vi "FPGA_controller.vi"() -> ()   [LabVIEW 2017]
uses:
  <vilib>/rvi/Emulation/niFpgaGetClockAttributes.vi
  <vilib>/rvi/Emulation/niFpgaSctlEmulationGetInTimedLoop.vi
  <vilib>/rvi/Emulation/niFpgaEmulationReportErrorSimple.vi
  <vilib>/rvi/eio/common/nirviEmuTemplateMethod_errors.vi
  <vilib>/rvi/Emulation/niFpgaCriticalErrorInLSC.vi
  <vilib>/eio/EIONode/EIONode.xnode
panel:
  out "Translated":i16
  out "VALID":bool
  in  "m_first u2":fxp<+/-,64,32>=-0.8999999999068677 format="%#_42g"
  in  "m_first u1":fxp<+/-,64,32>=-0.8999999999068677 format="%#_42g"
  in  "Scale u2":fxp<+/-,64,42>=5.0 format="%#_35g"
  in  "Offset u2":fxp<+/-,64,41>=2.0 format="%#_36g"
  in  "Scale u1":fxp<+/-,64,42>=5.0 format="%#_35g"
  in  "Offset u1":fxp<+/-,64,41>=2.0 format="%#_36g"
  in  "eta u":fxp<+/-,64,32>=0.30000000004656613 format="%#_42g"
  in  "Scale x2":fxp<+/-,32,16>=10.0 format="%#_21g"
  in  "m_first x2":fxp<+/-,49,33> format="%#_26g"
  in  "Offset x2":fxp<+/-,48,32> format="%#_26g"
  in  "Offset x3":fxp<+/-,48,32>=5.0 format="%#_26g"
  in  "m_first x3":fxp<+/-,32,16>=-3.399993896484375 format="%#_21g"
  in  "Scale x3":fxp<+/-,32,16>=10.0 format="%#_21g"
  in  "1/eta x":fxp<+/-,32,16>=5.0 format="%#_21g"
  in  "m_first x1":fxp<+/-,49,33> format="%#_26g"
  in  "Offset x1":fxp<+/-,48,32> format="%#_26g"
  in  "Scale x1":fxp<+/-,32,16>=10.0 format="%#_21g"
  in  "stop":bool
  # "INPUTS CONVERSION"
  # "STATES CONVERSION"
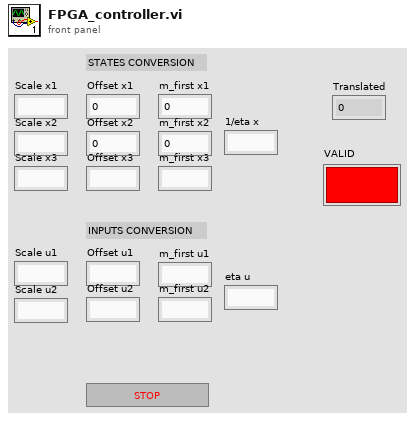
[diagram p1: front panel]
types:
  T1 = cluster{"Boolean array[0]":bool, "Boolean array[1]":bool, "Boolean array[2]":bool, "Boolean array[3]":bool, "Boolean array[4]":bool, "Boolean array[5]":bool, "Boolean array[6]":bool, "Boolean array[7]":bool, "Boolean array[8]":bool, "Boolean array[9]":bool, "Boolean array[10]":bool, "Boolean array[11]":bool, "Boolean array[12]":bool, "Boolean array[13]":bool, "Boolean array[14]":bool, "Boolean array[15]":bool, "Boolean array[16]":bool, "Boolean array[17]":bool}
  T2 = cluster{"Boolean array[0]":bool, "Boolean array[1]":bool, "Boolean array[2]":bool, "Boolean array[3]":bool, "Boolean array[4]":bool, "Boolean array[5]":bool}
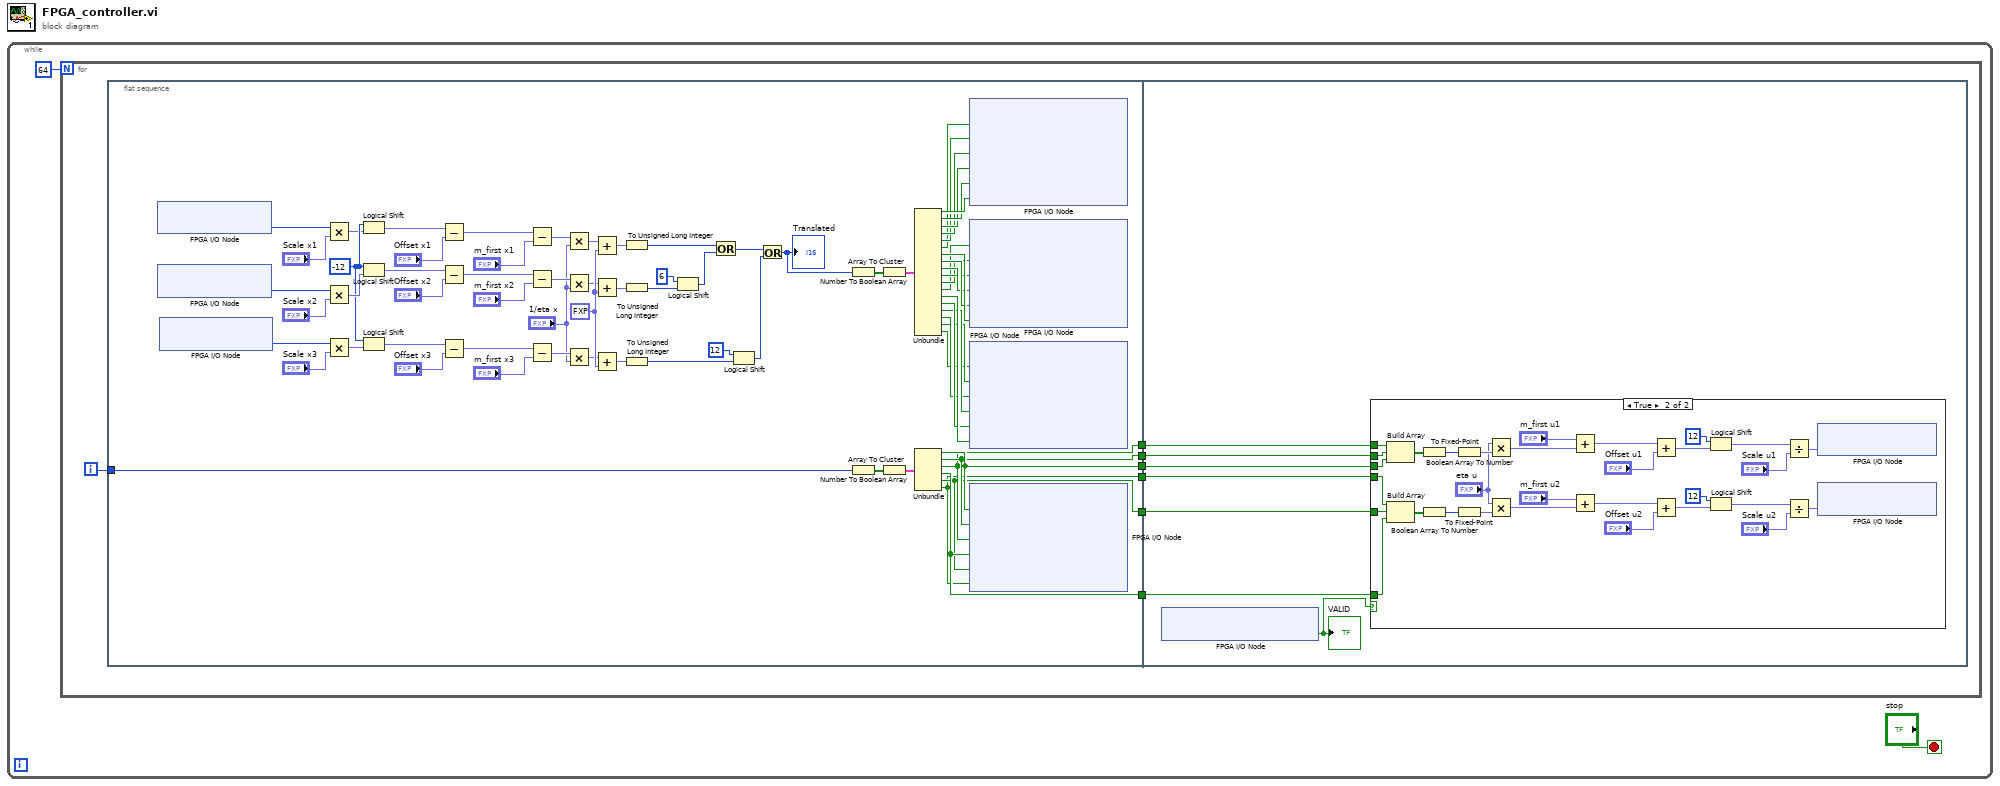
[diagram p0: block diagram]
diagram:
  n1 = while {
    stop <- "stop" stop-if-true
    n2 = for {
      N: 64 -> [_]
      i -> [w9]
      n3 = flat-sequence {
        tunnel: w9 -> [w79]
        tunnel: [w77] -> w8
        tunnel: [w76] -> w7
        tunnel: [w75] -> w6
        tunnel: [w74] -> w5
        tunnel: [w73] -> w4
        tunnel: [w72] -> w3
        tunnel: w8 -> [w87]
        tunnel: w7 -> [w86]
        tunnel: w6 -> [w85]
        tunnel: w5 -> [w84]
        tunnel: w4 -> [w83]
        tunnel: w3 -> [w82]
        frame #0 {
          w41 = fxp<+/-,64,32> 0.5 ("y")
          w36 = i16 -12 ("y")
          n4 = xnode "FPGA I/O Node"() -> ("ConnectorA/AI0"=w30:u16)  [unwired: 1 in, 1 out]
          n5 = xnode "FPGA I/O Node"() -> ("ConnectorA/AI1"=w35:u16)  [unwired: 1 in, 1 out]
          n6 = xnode "FPGA I/O Node"() -> ("ConnectorB/AI0"=w34:u16)  [unwired: 1 in, 1 out]
          n7 = Multiply(x=w30, y="Scale x1") -> (x*y=w29:fxp<+/-,48,32>)
          n8 = Multiply(x=w35, y="Scale x2") -> (x*y=w42:fxp<+/-,48,32>)
          n9 = Multiply(x=w34, y="Scale x3") -> (x*y=w32:fxp<+/-,48,32>)
          n10 = Logical Shift(y=w36, x=w29) -> (x << y=w26:fxp<+/-,48,32>)
          n11 = Logical Shift(y=w36, x=w42) -> (x << y=w23:fxp<+/-,48,32>)
          n12 = Logical Shift(y=w36, x=w32) -> (x << y=w31:fxp<+/-,48,32>)
          n13 = Subtract(x=w26, y="Offset x1") -> (x-y=w27:fxp<+/-,49,33>)
          n14 = Subtract(x=w23, y="Offset x2") -> (x-y=w24:fxp<+/-,49,33>)
          n15 = Subtract(x=w31, y="Offset x3") -> (x-y=w33:fxp<+/-,49,33>)
          n16 = Subtract(x=w27, y="m_first x1") -> (x-y=w28:fxp<+/-,50,34>)
          n17 = Subtract(x=w24, y="m_first x2") -> (x-y=w22:fxp<+/-,50,34>)
          n18 = Subtract(x=w33, y="m_first x3") -> (x-y=w38:fxp<+/-,50,34>)
          n19 = Multiply(x=w28, y="1/eta x") -> (x*y=w25:fxp<+/-,64,49>)
          n20 = Multiply(x=w22, y="1/eta x") -> (x*y=w21:fxp<+/-,64,49>)
          n21 = Multiply(x=w38, y="1/eta x") -> (x*y=w37:fxp<+/-,64,49>)
          n22 = Add(x=w25, y=w41) -> (x+y=w51:fxp<+/-,64,50>)
          n23 = Add(x=w21, y=w41) -> (x+y=w40:fxp<+/-,64,50>)
          n24 = Add(x=w37, y=w41) -> (x+y=w39:fxp<+/-,64,50>)
          n25 = To Unsigned Long Integer(number=w51) -> (unsigned 32bit integer=w47:u32)
          n26 = To Unsigned Long Integer(number=w40) -> (unsigned 32bit integer=w49:u32)
          n27 = To Unsigned Long Integer(number=w39) -> (unsigned 32bit integer=w45:u32)
          n28 = Logical Shift(y=6, x=w49) -> (x << y=w48:u32)
          n29 = Or(x=w47, y=w48) -> (x .or. y?=w43:u32)
          n30 = Logical Shift(y=12, x=w45) -> (x << y=w44:u32)
          n31 = Or(x=w43, y=w44) -> (x .or. y?=w10:u32)
          "Translated" <- w10
          n32 = Number To Boolean Array(number=w10) -> (Boolean array=w52:bool[])
          n33 = Number To Boolean Array(number=w79) -> (Boolean array=w80:bool[])
          n34 = Array To Cluster(array=w52) -> (cluster=w71:T1)
          n35 = Array To Cluster(array=w80) -> (cluster=w78:T2)
          n36 = Unbundle(w71) -> ("Boolean array[0]"=w70:bool, "Boolean array[1]"=w69:bool, "Boolean array[2]"=w68:bool, "Boolean array[3]"=w67:bool, "Boolean array[4]"=w66:bool, "Boolean array[5]"=w65:bool, "Boolean array[6]"=w64:bool, "Boolean array[7]"=w63:bool, "Boolean array[8]"=w62:bool, "Boolean array[9]"=w61:bool, "Boolean array[10]"=w60:bool, "Boolean array[11]"=w59:bool, "Boolean array[12]"=w58:bool, "Boolean array[13]"=w57:bool, "Boolean array[14]"=w56:bool, "Boolean array[15]"=w55:bool, "Boolean array[16]"=w54:bool, "Boolean array[17]"=w53:bool)
          n37 = Unbundle(w78) -> ("Boolean array[0]"=w77:bool, "Boolean array[1]"=w76:bool, "Boolean array[2]"=w75:bool, "Boolean array[3]"=w74:bool, "Boolean array[4]"=w73:bool, "Boolean array[5]"=w72:bool)
          n38 = xnode "FPGA I/O Node"("Component-Level IP\\pi00"=w65, "Component-Level IP\\pi01"=w66, "Component-Level IP\\pi02"=w67, "Component-Level IP\\pi03"=w68, "Component-Level IP\\pi04"=w69, "Component-Level IP\\pi05"=w70) -> ()  [unwired: 6 in, 6 out]
          n39 = xnode "FPGA I/O Node"("Component-Level IP\\pi06"=w59, "Component-Level IP\\pi07"=w60, "Component-Level IP\\pi08"=w61, "Component-Level IP\\pi09"=w62, "Component-Level IP\\pi10"=w63, "Component-Level IP\\pi11"=w64) -> ()  [unwired: 6 in, 6 out]
          n40 = xnode "FPGA I/O Node"("Component-Level IP\\pi12"=w53, "Component-Level IP\\pi13"=w54, "Component-Level IP\\pi14"=w55, "Component-Level IP\\pi15"=w56, "Component-Level IP\\pi16"=w57, "Component-Level IP\\pi17"=w58) -> ()  [unwired: 6 in, 6 out]
          n41 = xnode "FPGA I/O Node"("Component-Level IP\\pi18"=w77, "Component-Level IP\\pi19"=w76, "Component-Level IP\\pi20"=w75, "Component-Level IP\\pi21"=w74, "Component-Level IP\\pi22"=w73, "Component-Level IP\\pi23"=w72) -> ()  [unwired: 6 in, 6 out]
        }
        frame #1 {
          n42 = xnode "FPGA I/O Node"() -> ("Component-Level IP\\po0"=w81:bool)  [unwired: 1 in, 1 out]
          "VALID" <- w81
          n43 = case shown="True" w81 {
            tunnel: w87 -> [_ w100]
            tunnel: w86 -> [_ w99]
            tunnel: w85 -> [_ w98]
            tunnel: w84 -> [_ w97]
            tunnel: w83 -> [_ w96]
            tunnel: w82 -> [_ w95]
            frame False {
            }
            frame True {
              n44 = Build Array(w98, w99, w100) -> (w117:bool[])
              n45 = Build Array(w95, w96, w97) -> (w108:bool[])
              n46 = Boolean Array To Number(Boolean array=w117) -> (number=w115:u8)
              n47 = Boolean Array To Number(Boolean array=w108) -> (number=w106:u8)
              n48 = To Fixed-Point(number=w115) -> (fixed-point=w114:fxp<+,8,8>)  [unwired: 1 in]
              n49 = To Fixed-Point(number=w106) -> (fixed-point=w105:fxp<+,8,8>)  [unwired: 1 in]
              n50 = Multiply(x="eta u", y=w114) -> (x*y=w118:fxp<+/-,64,40>)
              n51 = Multiply(x="eta u", y=w105) -> (x*y=w109:fxp<+/-,64,40>)
              n52 = Add(x="m_first u1", y=w118) -> (x+y=w116:fxp<+/-,64,41>)
              n53 = Add(x="m_first u2", y=w109) -> (x+y=w107:fxp<+/-,64,41>)
              n54 = Add(x=w116, y="Offset u1") -> (x+y=w113:fxp<+/-,64,42>)
              n55 = Add(x=w107, y="Offset u2") -> (x+y=w104:fxp<+/-,64,42>)
              n56 = Logical Shift(y=i16 12, x=w113) -> (x << y=w111:fxp<+/-,64,42>)
              n57 = Logical Shift(y=i16 12, x=w104) -> (x << y=w102:fxp<+/-,64,42>)
              n58 = Divide(x=w111, y="Scale u1") -> (x/y=w110:fxp<+/-,64,65>)
              n59 = Divide(x=w102, y="Scale u2") -> (x/y=w101:fxp<+/-,64,65>)
              n60 = xnode "FPGA I/O Node"("ConnectorB/AO0"=w110) -> ()  [unwired: 1 in, 1 out]
              n61 = xnode "FPGA I/O Node"("ConnectorB/AO1"=w101) -> ()  [unwired: 1 in, 1 out]
            }
          }
        }
      }
    }
  }
